vi "Get_Status.vi"(1 "Status Array":T1(array[cluster]), 2 "Event":cluster{string, string[], dbl[], dbl}) -> (0 "Status":string)   [LabVIEW 2011]
doc: "This VI looks up the \"Status\" for a given event in the \"Status Array\". The \"Status\" string is typically a simple line of text informing the growth sequence operator of any values or readings updated by the given event."
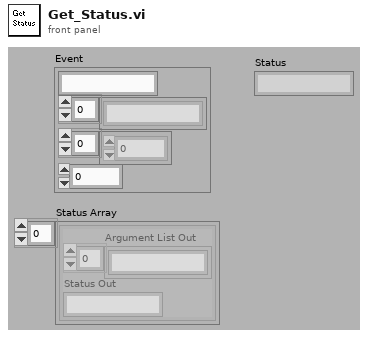
[diagram p1: front panel]
types:
  T1 = cluster{"Argument List Out":string[], "Status Out":string}[]
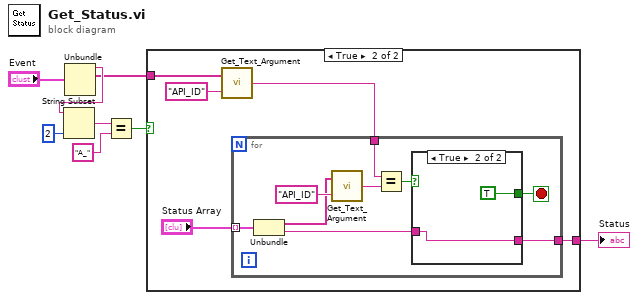
[diagram p0: block diagram]
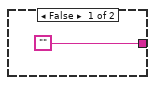
[diagram p2: hidden frame]
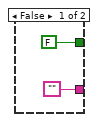
[diagram p3: hidden frame]
diagram:
  n1 = Unbundle("Event") -> (w8:string, w1:string[])  [unwired: 2 out]
  n2 = String Subset(string=w8, length (rest)=2 ("length (rest)")) -> (substring=w6:string)  [unwired: 1 out]
  n3 = Equal?(x=w6, y="A_") -> (x = y?=w3:bool)
  n4 = case shown="True" w3 {
    tunnel: ["" w14] -> w2
    tunnel: w1 -> [_ w12]
    frame False {
    }
    frame True {
      n5 = call "Get_Text_Argument.vi"("Argument"="API_ID", "Argument List"=w12) -> ("Text"=w10:string)
      n6 = for {
        tunnel: "Status Array" -> [w23] mode=indexing
        tunnel: [w17] -> w14
        tunnel: w10 -> [w19]
        stop <- w15 stop-if-true
        n7 = Unbundle(w23) -> ("Argument List Out"=w21:string[], "Status Out"=w16:string)
        n8 = call "Get_Text_Argument.vi"("Argument"="API_ID", "Argument List"=w21) -> ("Text"=w20:string)
        n9 = Equal?(x=w19, y=w20) -> (x = y?=w18:bool)
        n10 = case shown="True" w18 {
          tunnel: ["" w27] -> w17
          tunnel: w16 -> [_ w27]
          tunnel: [FALSE TRUE] -> w15
          frame False {
          }
          frame True {
          }
        }
      }
    }
  }
  "Status" <- w2
